vi "Exploring data entry 2.vi"() -> ()   [LabVIEW 2015]
uses:
  <vilib>/Utility/miscctls.llb/LVRowAndColumnTypeDef.ctl
panel:
  in  "Product":dbl(ring) items=["Select...", "One", "Two", "Three", "Four"]
  in  "Amount":dbl=10.0 min=0.0
  out "Table Indicator":string[][](table)=[["Select...", "0.00", "This Week", "0.0", "0", "0", "0", "0", "0", "0", "0", "0"], ["Select...", "0.00", "This Week", "0.0", "0", "0", "0", "0", "0", "0", "0", "0"], ["Select...", "0.00", "This Week", "0.0", "0", "0", "0", "0", "0", "0", "0", "0"], ["Select...", "0.00", "This Week", "0.0", "0", "0", "0", "0", "0", "0", "0", "0"], ["Select...", "0.00", "This Week", "0.0", "0", "0", "0", "0", "0", "0", "0", "0"], ["Select...", "0.00", "This Week", "0.0", "0", "0", "0", "0", "0", "0", "0", "0"], ["Select...", "0.00", "This Week", "0.0", "0", "0", "0", "0", "0", "0", "0", "0"], ["Select...", "0.00", "This Week", "0.0", "0", "0", "0", "0", "0", "0", "0", "0"], ["Select...", "0.00", "This Week", "0.0", "0", "0", "0", "0", "0", "0", "0", "0"], ["Select...", "0.00", "This Week", "0.0", "0", "0", "0", "0", "0", "0", "0", "0"], ["Total", "", "", "0", "0", "0", "0", "0", "0", "0", "0", ""]]
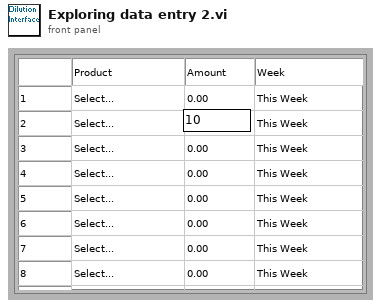
[diagram p1: front panel]
types:
  T1 = typedef "LVRowAndColumnTypeDef.ctl" = cluster{"Row":i32, "Column":i32}
  T2 = cluster{"Amount":dbl, "Amount 2":dbl, "Amount 3":dbl}
  T3 = cluster{"Amount":dbl, "Amount 2":dbl, "Amount 3":dbl}[]
  T4 = typedef "LVPoint32TypeDef.ctl" = cluster{"Horizontal":i32, "Vertical":i32}
  T5 = typedef "LVPositionTypeDef.ctl" = cluster{"Left":i32, "Top":i32}
  T6 = typedef "LVBoundsTypeDef.ctl" = cluster{"Width":u32, "Height":u32}
  T7 = typedef "LVFontTypeDef.ctl" = cluster{"Font Name":string, "Size":u16, "Bold":bool, "Italic":bool, "Underline":bool, "Strikeout":bool, "Color":u32}
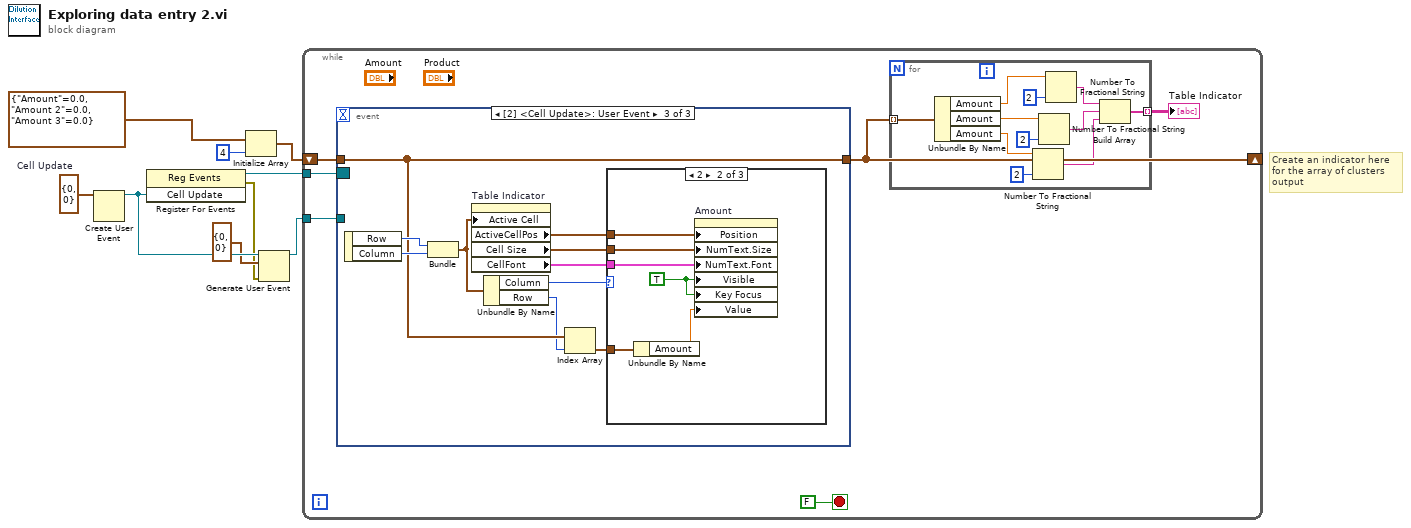
[diagram p0: block diagram]
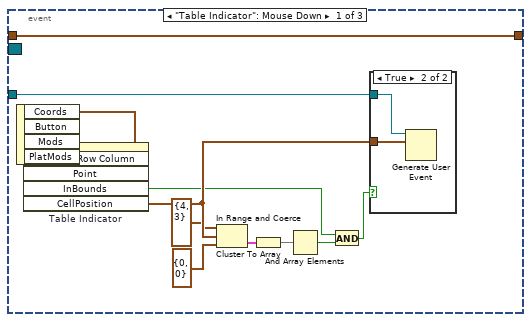
[diagram p2: hidden frame]
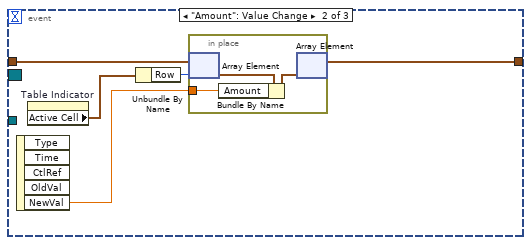
[diagram p4: hidden frame]
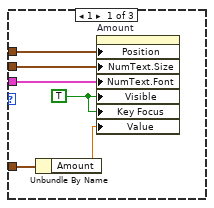
[diagram p5: hidden frame]
diagram:
  w7 = T1 {"Row"=0, "Column"=0}  # Cell Update
  # "Create an indicator here\nfor the array of clusters\noutput"
  n1 = Create User Event(user event datatype=w7) -> (user event=w4:refnum<user-event>)  [unwired: 1 in, 1 out]
  n2 = register-events(w4) -> (reference out=w6:refnum<event-registration>, error out=w2:errorcluster)  [unwired: 2 in]
  n3 = Initialize Array(T2 {"Amount"=0.0, "Amount 2"=0.0, "Amount 3"=0.0} ("Dilution Product Selection"), 4 ("dimension size")) -> (w8:T3)
  n4 = Generate User Event(user event=w4, event data cluster=T1 {"Row"=0, "Column"=0} ("event data"), error in=w2) -> (user event out=w1:refnum<user-event>)  [unwired: 1 in, 1 out]
  n5 = while {
    shift-right: [w13] -> _
    shift-left: w8 -> [w15]
    tunnel: w6 -> [w14]
    tunnel: w1 -> [w12]
    stop <- FALSE stop-if-true
    n6 = event shown="[2] <Cell Update>: User Event" {
      selector: w14 -> [_ _ _]
      dyn-events: _ -> [_ _ _]
      timeout: _ -> [_ _ _]
      tunnel: w15 -> [w28 w44 w50]
      tunnel: [w28 w42 w50] -> w13
      tunnel: w12 -> [w27 _ _]
      event "Table Indicator": Mouse Down {
        n7 = event-data() -> ("Coords"=w37:T4)  [unwired: 1 in, 3 out]
        n8 = invoke on="Table Indicator" class="Tbl (strict)" method="Point To Row Column"("Point"=w37) -> ("InBounds"=w32:bool, "CellPosition"=w36:T1)  [unwired: 5 in, 4 out]
        n9 = In Range and Coerce(upper limit=T1 {"Row"=4, "Column"=3}, x=w36, lower limit=T1 {"Row"=0, "Column"=0}) -> (In Range?=w33:cluster{"Row":bool, "Column":bool})  [unwired: 1 out]
        n10 = Cluster To Array(cluster=w33) -> (array=w30:bool[])
        n11 = And Array Elements(Boolean array=w30) -> (logical AND=w29:bool)
        n12 = And(x=w32, y=w29) -> (x .and. y?=w31:bool)
        n13 = case shown="True" w31 {
          tunnel: w36 -> [_ w39]
          tunnel: w27 -> [_ w38]
          frame False {
          }
          frame True {
            n14 = Generate User Event(user event=w38, event data cluster=w39) -> ()  [unwired: 2 in, 2 out]
          }
        }
      }
      event "Amount": Value Change {
        n15 = event-data() -> ("NewVal"=w41:dbl)  [unwired: 1 in, 4 out]
        n16 = property on="Table Indicator" class="Tbl (strict)"() -> ("Active Cell"=w40:T1)  [unwired: 2 in, 2 out]
        n17 = Unbundle By Name(w40) -> ("Row"=w43:i32)
        n18 = in-place {
          in-place-border: w41 -> [w45]
          n19 = in-place-array #1(w44, w43) -> (w47:T2)
          n20 = Bundle By Name(cluster=w47, "Amount"=w45) -> (w46:T2)
          n21 = in-place-array #1(w46) -> (w42:T3)  [unwired: 1 out]
        }
      }
      event User Event {
        n22 = event-data() -> ("Row"=w57:i32, "Column"=w56:i32)  [unwired: 1 in]
        n23 = Bundle("Row"=w57, "Column"=w56) -> (w51:cluster{"Row":i32, "Column":i32})  [unwired: 1 in]
        n24 = property on="Table Indicator" class="Tbl (strict)"("Active Cell"=w51) -> ("ActiveCellPos"=w55:T5, "Cell Size"=w54:T6, "CellFont"=w52:T7)  [unwired: 2 in, 2 out]
        n25 = Unbundle By Name(w51) -> ("Column"=w53:i32, "Row"=w49:i32)
        n26 = Index Array(array=w50, index=w49) -> (element=w48:T2)
        n27 = case shown="2" w53 {
          tunnel: w55 -> [w63 w69 _]
          tunnel: w54 -> [w62 w68 _]
          tunnel: w52 -> [w60 w66 _]
          tunnel: w48 -> [w59 w65 _]
          frame 1 {
            w61 = TRUE ("Key Focus")
            n28 = Unbundle By Name(w59) -> ("Amount"=w58:dbl)
            n29 = property on="Amount" class="DigNum (strict)"("Position"=w63, "NumText.Size"=w62, "NumText.Font"=w60, "Visible"=w61, "Key Focus"=w61, "Value"=w58) -> ()  [unwired: 2 in, 2 out]
          }
          frame 2 {
            w67 = TRUE ("Key Focus")
            n30 = Unbundle By Name(w65) -> ("Amount"=w64:dbl)
            n31 = property on="Amount" class="DigNum (strict)"("Position"=w69, "NumText.Size"=w68, "NumText.Font"=w66, "Visible"=w67, "Key Focus"=w67, "Value"=w64) -> ()  [unwired: 2 in, 2 out]
          }
          frame Default {
          }
        }
      }
    }
    n32 = for {
      tunnel: [w23] -> w11 mode=indexing
      tunnel: w13 -> [w22] mode=indexing
      n33 = Unbundle By Name(w22) -> ("Amount"=w20:dbl, "Amount"=w26:dbl, "Amount"=w16:dbl)
      n34 = Number To Fractional String(number=w16, precision (6)=i16 2) -> (F-format string=w17:string)  [unwired: 2 in]
      n35 = Number To Fractional String(number=w26, precision (6)=i16 2) -> (F-format string=w25:string)  [unwired: 2 in]
      n36 = Number To Fractional String(number=w20, precision (6)=i16 2) -> (F-format string=w19:string)  [unwired: 2 in]
      n37 = Build Array(w19, w25, w17) -> (w23:string[])
    }
    "Table Indicator" <- w11
  }
